vi "GetDebugImage.vi"(2 "image":T1, 3 "tracker":u64) -> (0 "image":T1(plugin-control), 1 "tracker":u64)   [LabVIEW 2011]
uses:
  <vilib>/vision/Image Controls.llb/IMAQ Image.ctl
  TrackerDLL.vi
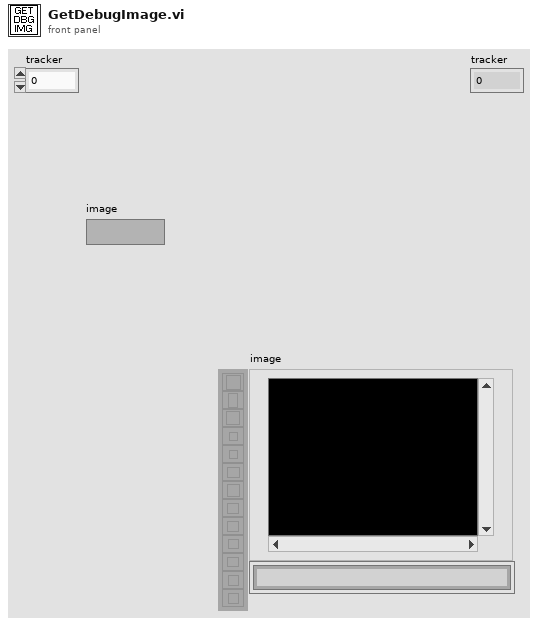
[diagram p1: front panel]
types:
  T1 = typedef "IMAQ Image.ctl" = refnum<image>
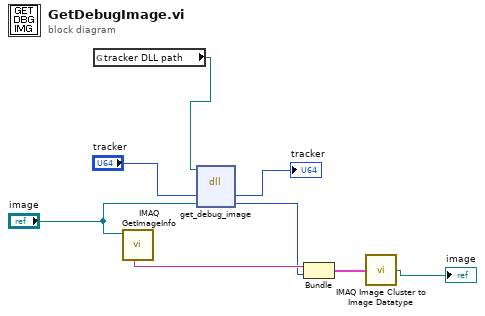
[diagram p0: block diagram]
diagram:
  n1 = global read "TrackerDLL.vi" "tracker DLL path"() -> (w8:path)
  n2 = call "IMAQ GetImageInfo"("Image"="image") -> ("Image Name"=w3:string)  [unwired: 3 in, 7 out]
  n3 = dll-call lib="D:/jcnossen1/cudaqi-tracker/cudatrack-labview/cputrack.dll" fn="get_debug_image"(path in=w8, "tracker"="tracker", "image"="image") -> ("tracker"=→"tracker":u64, "image"=w2:u64)  [unwired: 3 in, 2 out]
  n4 = Bundle("Image Name"=w3, "image"=w2) -> (w5:cluster{"Image Name":string, "image":u64})  [unwired: 1 in]
  n5 = call <vilib>:"IMAQ Image Cluster to Image Datatype.vi"("Image"=w5) -> ("Image (dup)"=→"image":T1)
